vi "Send SMS simplified.vi"(3 "Message":string="This is a test massage", 4 "Subject":string="Testing", 5 "Carrier":string(combo)="@tmomail.net", 6 "Phone number":string="2816302191") -> (0 "Error Out":errorcluster, 2 "Invalid Recipients":string)   [LabVIEW 2018]
uses:
  <vilib>/smtpClient/Set Message Text.vi
  <vilib>/smtpClient/LabVIEWSMTPClient.lvlib
panel:
  in  "Error In":errorcluster
  in  "Port":string="587"
  in  "Sender email":string="kundulab270@gmail.com"
  in  "Username":string="kundulab270@gmail.com"
  in  "Password":string="xhjldkvdpmnzmmfe"
  in  "SMTP server":string="smtp.gmail.com"
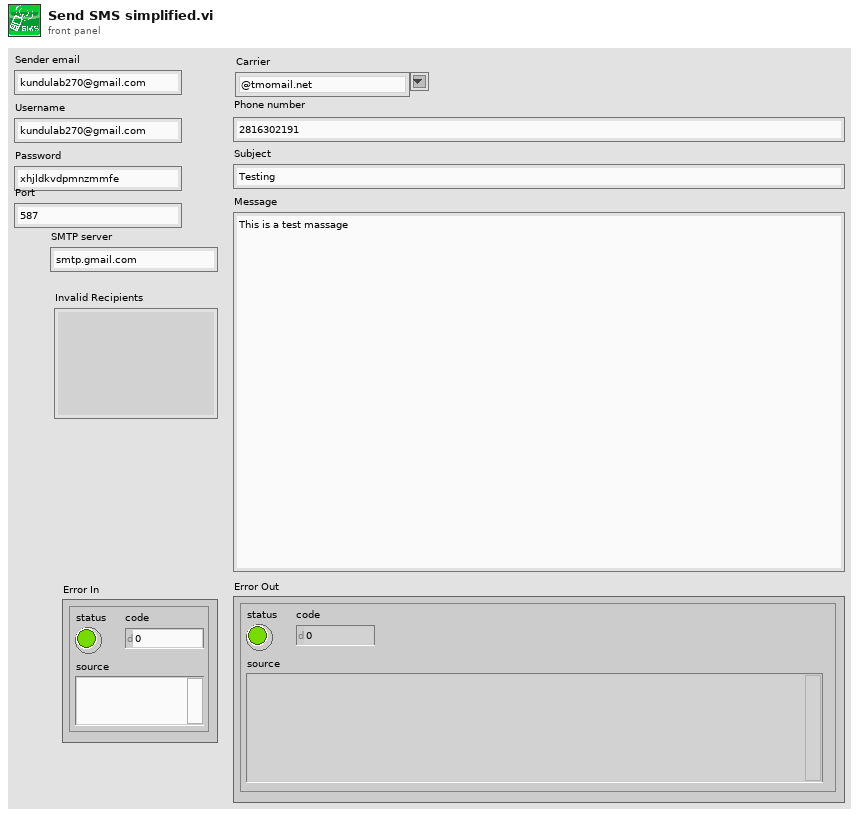
[diagram p1: front panel]
types:
  T1 = typedef "LabVIEWSMTPClient.lvlib/SmtpClientHandle.ctl" = refnum<k1>
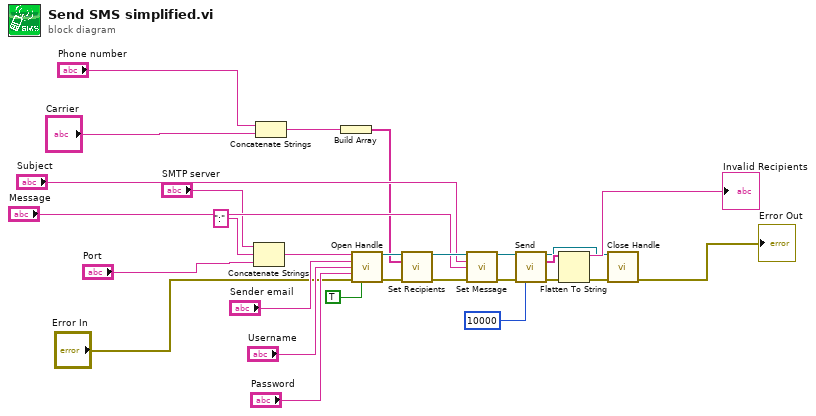
[diagram p0: block diagram]
diagram:
  n1 = Concatenate Strings("SMTP server", ":" ("string"), "Port") -> (w7:string)
  n2 = Concatenate Strings("Phone number", "Carrier") -> (w5:string)
  n3 = Build Array(w5) -> (w4:string[])
  n4 = call <vilib>:"Open Handle.vi"("server address"=w7, "from"="Sender email", "username"="Username", "password"="Password", "error in (no error)"="Error In", "use TLS (false)"=TRUE) -> ("handle out"=w17:T1, "error out"=w15:errorcluster)  [unwired: 8 in]
  n5 = call <vilib>:"Set Recipients.vi"("handle in"=w17, "to"=w4, "error in (no error)"=w15) -> ("handle out"=w18:T1, "error out"=w16:errorcluster)  [unwired: 11 in]
  n6 = call-poly <vilib>:"Set Message.vi"("handle in"=w18, "subject"="Subject", "plain text message"="Message", "error in (no error)"=w16) -> ("handle out"=w20:T1, "error out"=w19:errorcluster)  [unwired: 10 in]
  n7 = call <vilib>:"Send.vi"("handle in"=w20, "error in (no error)"=w19, "timeout in ms (10000)"=10000 ("timeout in ms")) -> ("handle out"=w21:T1, "invalid recipients"=w23:string[], "error out"=w24:errorcluster)  [unwired: 10 in]
  n8 = Flatten To String(anything=w23, error in (no error)=w24) -> (data string=→"Invalid Recipients":string, error out=w25:errorcluster)  [unwired: 2 in, 1 out]
  n9 = call <vilib>:"Close Handle.vi"("handle in"=w21, "error in (no error)"=w25) -> ("error out"=→"Error Out":errorcluster)  [unwired: 12 in, 1 out]
